vi "Data_Read.vi"(0 "file (use dialog)":path, 1 "Data Read Count":i32=-1, 2 "Data Read Control":T1, 3 "error initialize":errorcluster) -> (6 "Read text":string, 7 "Read Cancelled":bool, 9 "error out":errorcluster)   [LabVIEW 2015]
uses:
  Data Read Control.ctl
panel:
  out "path":path
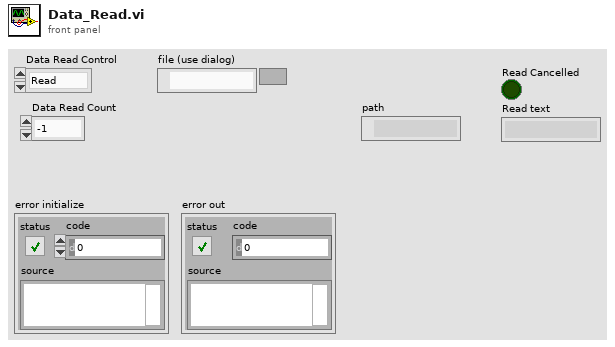
[diagram p1: front panel]
types:
  T1 = typedef "Data Read Control.ctl" = enum16{"Read", "Close"}
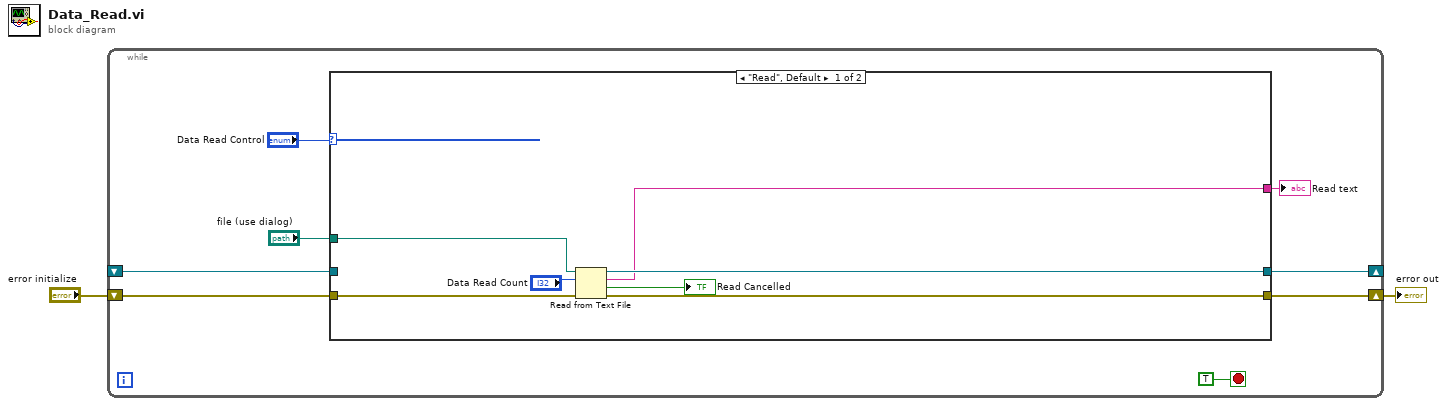
[diagram p0: block diagram]
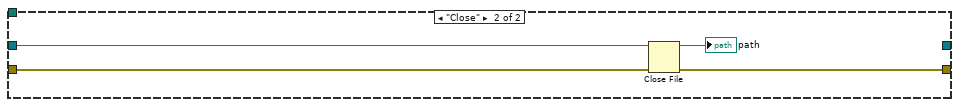
[diagram p2: hidden frame]
diagram:
  n1 = while {
    shift-right: [w9] -> w2
    shift-left: "error initialize" -> [w8]
    shift-right: [w7] -> _
    shift-left: _ -> [w6]
    stop <- TRUE stop-if-true
    n2 = case shown="\"Read\", Default" "Data Read Control" {
      tunnel: [w16 w21] -> w9
      tunnel: w8 -> [w17 w20]
      tunnel: [w15 _] -> w7
      tunnel: w6 -> [_ w19]
      tunnel: [w12 _] -> w4
      tunnel: "file (use dialog)" -> [w11 _]
      frame "Read", Default {
        n3 = Read from Text File(file (use dialog)=w11, count="Data Read Count", error in=w17) -> (refnum out=w15:refnum<file>, text=w12:string, cancelled=→"Read Cancelled":bool, error out=w16:errorcluster)  [unwired: 1 in]
      }
      frame "Close" {
        n4 = Close File(refnum=w19, error in=w20) -> (path=→"path":path, error out=w21:errorcluster)
      }
    }
    "Read text" <- w4
  }
  "error out" <- w2
